vi "Write F-I Map.vi"(8 "error in (no error)":errorcluster, 10 "F-I Map":map{string, refnum<class "Abs_Value.lvclass">}(c390), 11 "Fault-Injection Bus in":refnum<class "Fault-Injection Bus.lvclass">) -> (0 "error out":errorcluster, 3 "Fault-Injection Bus out":refnum<class "Fault-Injection Bus.lvclass">)   [LabVIEW 2021, in "Fault-Injection Bus.lvclass"]
uses:
  Fault-Injection Bus.lvclass
  Fault-Injection Bus.lvclass/Fault-Injection Bus.ctl
  <vilib>/TSA/Abstract Data Classes/Abs_Types/Value/Abs_Value.lvclass
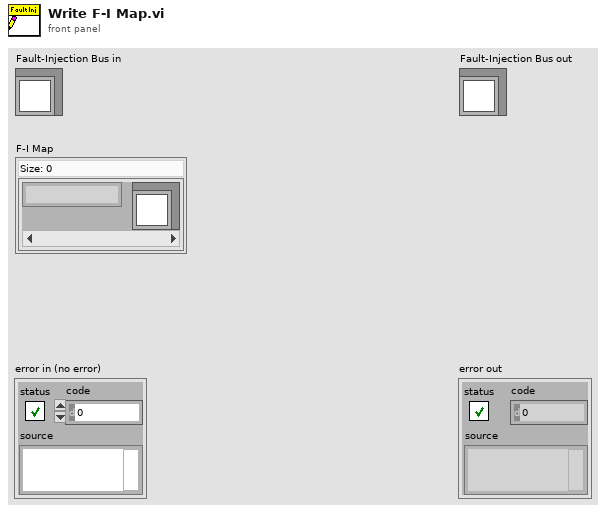
[diagram p1: front panel]
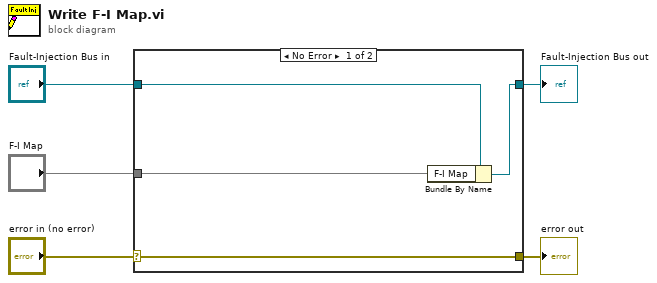
[diagram p0: block diagram]
diagram:
  n1 = case shown="No Error" "error in (no error)" {
    selector: "error in (no error)" -> [w9 w10]
    tunnel: [w9 w10] -> w4
    tunnel: [w7 w11] -> w2
    tunnel: "Fault-Injection Bus in" -> [w8 w11]
    tunnel: "F-I Map" -> [w6 _]
    frame No Error {
      n2 = Bundle By Name(cluster=w8, "F-I Map"=w6) -> (w7:refnum<class "Fault-Injection Bus.lvclass">)
    }
    frame Error {
    }
  }
  "error out" <- w4
  "Fault-Injection Bus out" <- w2
